vi "Calculate Accuracy.vi"(8 "error in (no error)":errorcluster, 11 "Calibration Points":T2[](array[typedef])) -> (0 "error out":errorcluster, 3 "Accuracy Results":T1[](array[typedef]))   [LabVIEW 2026, in "Analysis.lvlib"]
uses:
  Analysis.lvlib
  controls/Messaging Payloads/Calibration Point Table Insert.ctl
  Accuracy Result.ctl
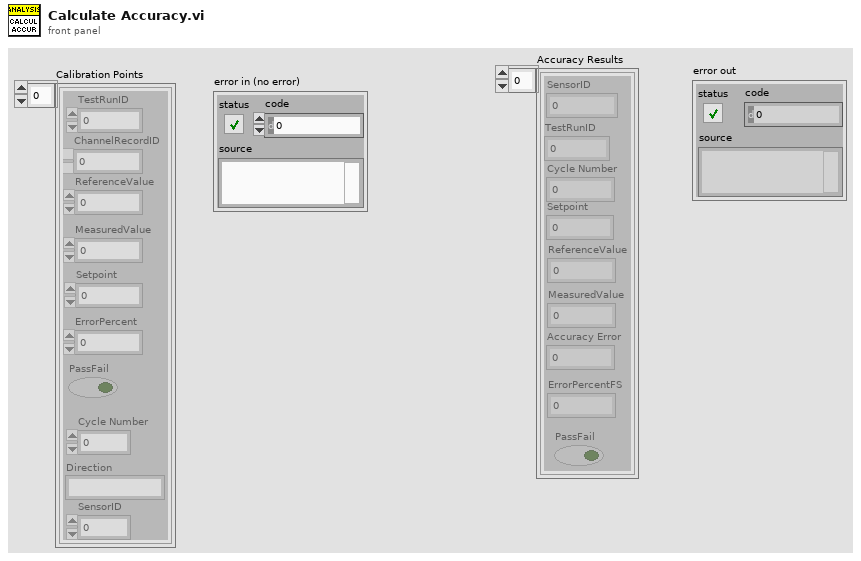
[diagram p1: front panel]
types:
  T1 = typedef "Analysis.lvlib/Accuracy Result.ctl" = cluster{"Setpoint":dbl, "Cycle Number":i32, "SensorID":i32, "TestRunID":i32, "ReferenceValue":dbl, "MeasuredValue":dbl, "ErrorPercentFS":dbl, "PassFail":bool, "Accuracy Error":dbl}
  T2 = typedef "Calibration Point Table Insert.ctl" = cluster{"TestRunID":i32, "ChannelRecordID":i32, "Setpoint":dbl, "MeasuredValue":dbl, "ErrorPercent":dbl, "PassFail":bool, "ReferenceValue":dbl, "Cycle Number":i32, "Direction":string, "SensorID":i32}
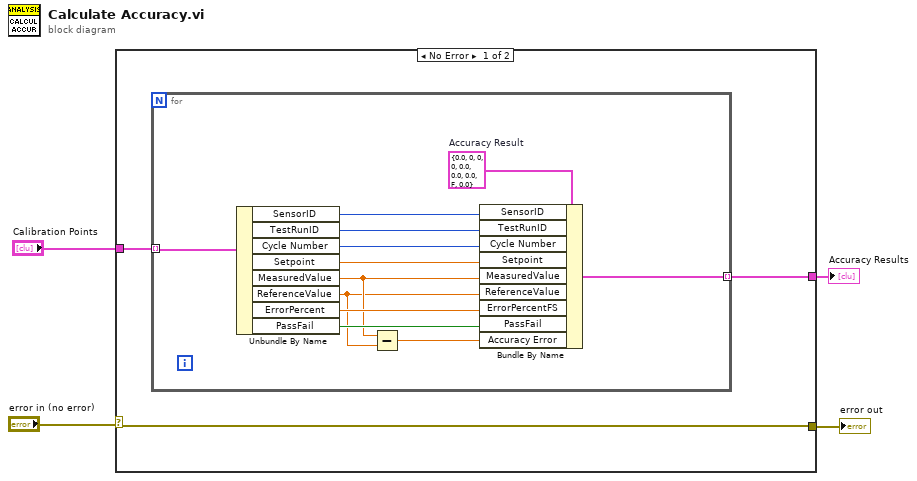
[diagram p0: block diagram]
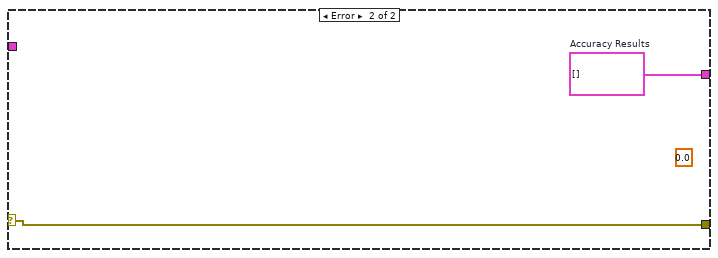
[diagram p2: hidden frame]
diagram:
  n1 = case shown="No Error" "error in (no error)" {
    selector: "error in (no error)" -> [w7 w21]
    tunnel: "Calibration Points" -> [w6 _]
    tunnel: [w7 w21] -> w2
    tunnel: [w5 w20] -> w1
    frame No Error {
      n2 = for {
        tunnel: w6 -> [w19] mode=indexing
        tunnel: [w9] -> w5 mode=indexing
        w18 = T1 {"Setpoint"=0.0, "Cycle Number"=0, "SensorID"=0, "TestRunID"=0, "ReferenceValue"=0.0, "MeasuredValue"=0.0, "ErrorPercentFS"=0.0, "PassFail"=FALSE, "Accuracy Error"=0.0}  # Accuracy Result
        n3 = Unbundle By Name(w19) -> ("SensorID"=w17:i32, "TestRunID"=w16:i32, "Cycle Number"=w15:i32, "Setpoint"=w14:dbl, "MeasuredValue"=w11:dbl, "ReferenceValue"=w10:dbl, "ErrorPercent"=w13:dbl, "PassFail"=w12:bool)
        n4 = Subtract(x=w11, y=w10) -> (x-y=w8:dbl)
        n5 = Bundle By Name(cluster=w18, "SensorID"=w17, "TestRunID"=w16, "Cycle Number"=w15, "Setpoint"=w14, "MeasuredValue"=w11, "ReferenceValue"=w10, "ErrorPercentFS"=w13, "PassFail"=w12, "Accuracy Error"=w8) -> (w9:T1)
      }
    }
    frame Error {
      (unwired) 0.0
      w20 = T1[] []  # Accuracy Results
    }
  }
  "error out" <- w2
  "Accuracy Results" <- w1
